vi "ExponentialMovingAverage.vi"(2 "old value":dbl=0.51444, 3 "current value":dbl=0.51444, 4 "weight":dbl=0.51444) -> (1 "average":dbl=0.51444)   [LabVIEW 2013]
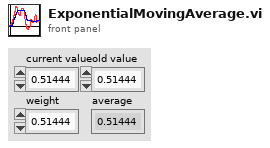
[diagram p1: front panel]
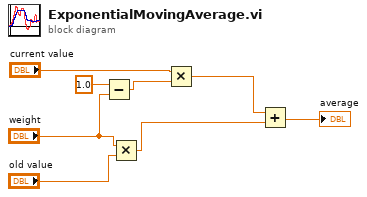
[diagram p0: block diagram]
diagram:
  n1 = Subtract(x=1.0, y="weight") -> (x-y=w4:dbl)
  n2 = Multiply(x="weight", y="old value") -> (x*y=w2:dbl)
  n3 = Multiply(x="current value", y=w4) -> (x*y=w3:dbl)
  n4 = Add(x=w3, y=w2) -> (x+y=→"average":dbl)
